vi "_TangoSetAttributeInfo.vi"(1 "error in":errorcluster, 2 "attribute info":T1={"device name"="", "attribute name"="", "r/w access"=enum."UNKNOWN_ACCESS_TYPE", "format"=enum."UNKNOWN_FORMAT", "data type"=enum."UNKNOW_DATA_TYPE", "level"=enum."UNKNOWN_LEVEL", "label"="", "unit"="", "display format"="", "min value"="", "max value"="", "min alarm"="", "max alarm"=""}) -> (0 "error out":errorcluster)   [LabVIEW 2014, in "tango.lvlib"]
uses:
  tango.lvlib
  Common VIs/Typedefs/_AttributeInfo_t.ctl
  Common VIs/Typedefs/_AttributeAccess_t.ctl
  Common VIs/Typedefs/_AttributeFormat_t.ctl
  Common VIs/Typedefs/_TangoDataType_t.ctl
  Common VIs/Typedefs/_AttributeLevel_t.ctl
  tango_binding.so
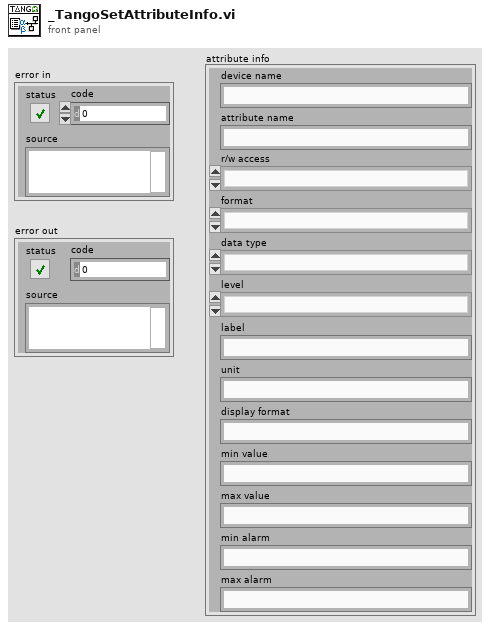
[diagram p1: front panel]
types:
  T1 = typedef "tango.lvlib/_AttributeInfo_t.ctl" = cluster{"device name":string, "attribute name":string, "r/w access":T2, "format":T3, "data type":T4, "level":T5, "label":string, "unit":string, "display format":string, "min value":string, "max value":string, "min alarm":string, "max alarm":string}
  T2 = typedef "tango.lvlib/_AttributeAccess_t.ctl" = enum16{"READ", "READ_WITH_WRITE", "WRITE", "READ_WRITE", "UNKNOWN_ACCESS_TYPE"}
  T3 = typedef "tango.lvlib/_AttributeFormat_t.ctl" = enum16{"SCALAR", "SPECTRUM", "IMAGE", "UNKNOWN_FORMAT"}
  T4 = typedef "tango.lvlib/_TangoDataType_t.ctl" = enum16{"VOID", "BOOLEAN", "SHORT", "LONG", "FLOAT", "DOUBLE", "USHORT", "ULONG", "STRING", "CHAR_ARRAY", "SHORT_ARRAY", "LONG_ARRAY", "FLOAT_ARRAY", "DOUBLE_ARRAY", "USHORT_ARRAY", "ULONG_ARRAY", "STRING_ARRAY", "LONG_STRING_ARRAY", "DOUBLE_STRING_ARRAY", "STATE", "CONST_STRING", "BOOLEAN_ARRAY", "UCHAR", "LONG64", "ULONG64", "LONG64_ARRAY", "ULONG64_ARRAY", "INT (not supported)", "ENCODED (not supported)", "ENUM", "PIPE_BLOB (not supported)", "STATE_ARRAY", "UNKNOW_DATA_TYPE"}
  T5 = typedef "tango.lvlib/_AttributeLevel_t.ctl" = enum16{"OPERATOR", "EXPERT", "UNKNOWN_LEVEL"}
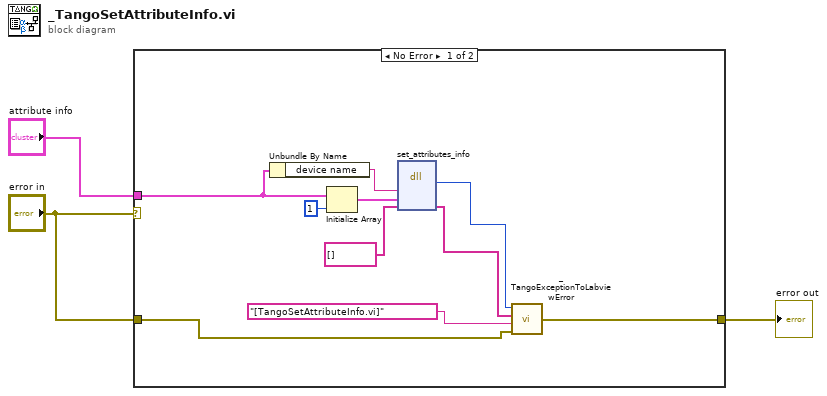
[diagram p0: block diagram]
diagram:
  n1 = case shown="No Error" "error in" {
    tunnel: [w12 w14] -> w2
    tunnel: "error in" -> [w11 w14]
    tunnel: "attribute info" -> [w4 _]
    frame No Error {
      n2 = Unbundle By Name(w4) -> ("device name"=w5:string)
      n3 = Initialize Array(w4, 1 ("dimension size")) -> (w8:T1[])
      n4 = dll-call lib="tango_binding.*" fn="set_attributes_info"("dev_name"=w5, "attrs_info_inout"=w8, "error_stack"=string[] [] ("error stack")) -> ("return type"=w6:i32, "error_stack"=w7:string[])  [unwired: 5 in, 2 out]
      n5 = call "_TangoExceptionToLabviewError.vi"("error in"=w11, "location"="[TangoSetAttributeInfo.vi]", "error stack"=w7, "error code"=w6) -> ("error out"=w12:errorcluster)
    }
    frame Error {
    }
  }
  "error out" <- w2
